vi "http connection handler.vi"(8 "http responder":refnum<class "http responder.lvclass">, 9 "remote address":string, 10 "basic HTTP handler dataset":refnum<class "basic HTTP handler dataset.lvclass">, 11 "connection":refnum<k5>) -> ()   [LabVIEW 2016, in "Basic HTTP server.lvclass"]
uses:
  Basic HTTP server.lvclass
  HTTP responder/http responder.lvclass
  HTTP handler dataset/basic HTTP handler dataset.lvclass
  http request.ctl
  http method.ctl
  HTTP headers/http header data.ctl
  http response.ctl
  http response packet type.ctl
  HTTP handler dataset/basic HTTP handler dataset.lvclass/basic HTTP handler dataset.ctl
  http parse state.ctl
  HTTP headers/http headers.lvlib
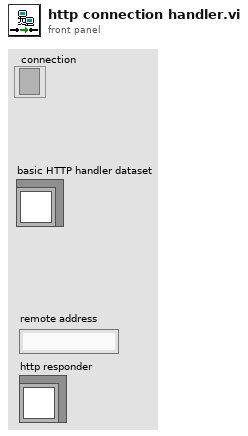
[diagram p1: front panel]
types:
  T1 = typedef "Basic HTTP server.lvclass/http response.ctl" = cluster{"packet type":T2, "reason code":u16, "status string":string, "headers":T3, "cookies":string[], "data":string}
  T2 = typedef "Basic HTTP server.lvclass/http response packet type.ctl" = enum16{"full response", "header only", "data only", "last data", "raw output"}
  T3 = typedef "http headers.lvlib/http header data.ctl" = cluster{"lookup":variant}
  T4 = typedef "Basic HTTP server.lvclass/http request.ctl" = cluster{"type":T5, "remote address":string, "method":string, "url":string, "version":string, "headers":T3, "data":string}
  T5 = typedef "Basic HTTP server.lvclass/http method.ctl" = enum16{"application", "error", "upgrade", "expect"}
  T6 = typedef "Basic HTTP server.lvclass/http server info.ctl" = cluster{"port":u16}
  T7 = typedef "Basic HTTP server.lvclass/http server properties.ctl" = cluster{"max url size":i32, "max header":i32, "timeout ms":i32, "max data size":i32}
  T8 = typedef "Basic HTTP server.lvclass/http parse state.ctl" = enum16{"function", "headers", "data"}
  T9 = enum16{"Standard", "Buffered", "CRLF", "Immediate"}
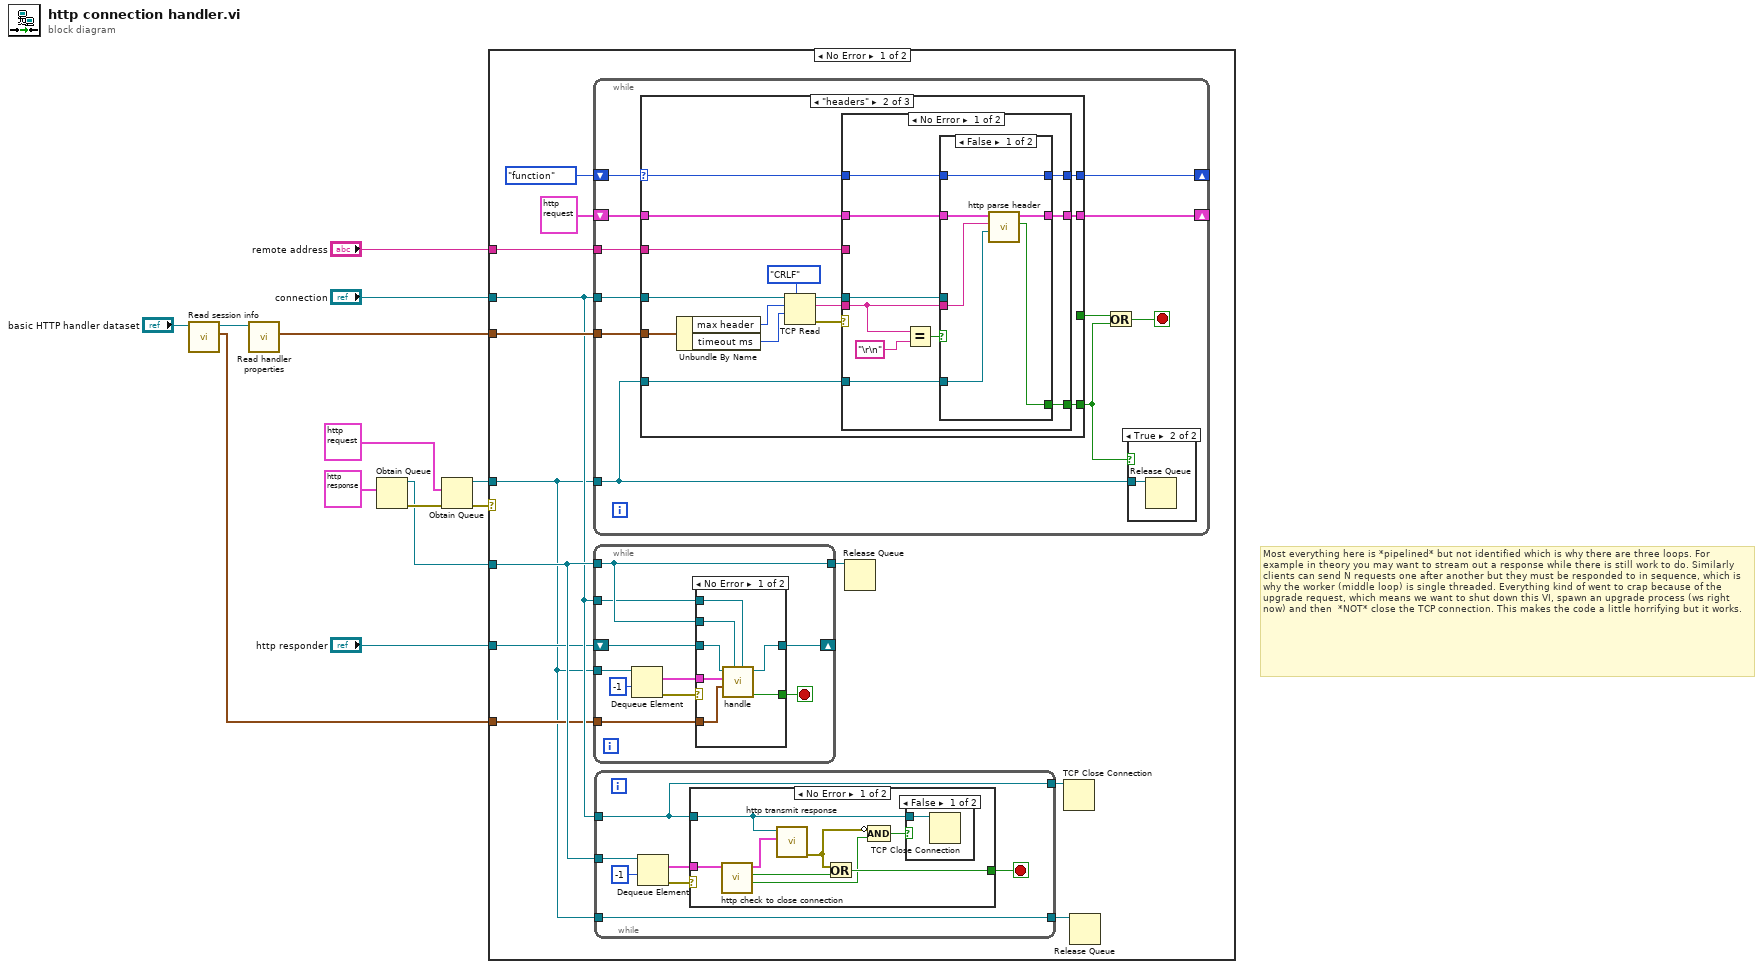
[diagram p0: block diagram]
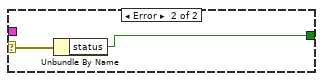
[diagram p3: hidden frame]
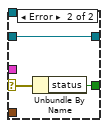
[diagram p4: hidden frame]
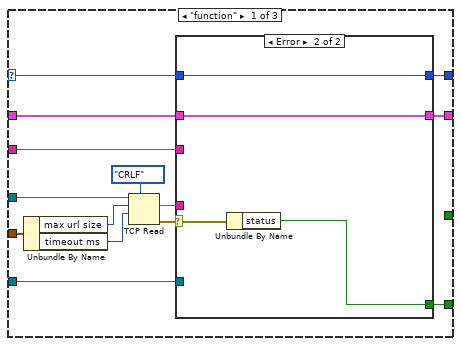
[diagram p6: hidden frame]
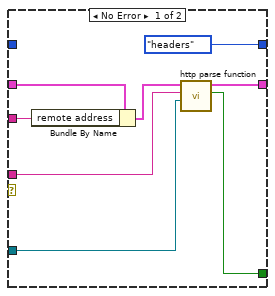
[diagram p7: hidden frame]
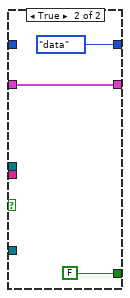
[diagram p8: hidden frame]
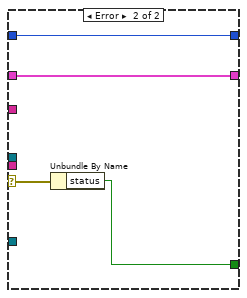
[diagram p9: hidden frame]
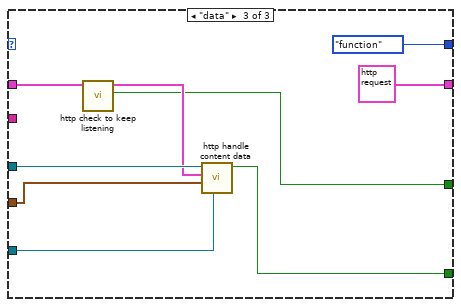
[diagram p10: hidden frame]
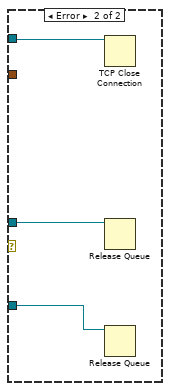
[diagram p11: hidden frame]
diagram:
  # "Most everything here is *pipelined* but not identified which is why there are three loops. For example in theory you may want to stream out a response while there is still work to do. Similarly clients can send N requests one after another but they must be responded to in sequence, which is why the worker (middle loop) is single threaded. Everything kind of went to crap because of the upgrade request, which means we want to shut down this VI, spawn an upgrade process (ws right now) and then  *NOT* close the TCP connection. This makes the code a little horrifying but it works."
  n1 = call "Read session info.vi"("basic HTTP handler dataset in"="basic HTTP handler dataset") -> ("server information"=w1:T6, "basic HTTP handler dataset out"=w2:refnum<class "basic HTTP handler dataset.lvclass">)  [unwired: 9 in]
  n2 = call "Read handler properties.vi"("basic HTTP handler dataset in"=w2) -> ("server properties"=w4:T7)  [unwired: 9 in, 1 out]
  n3 = Obtain Queue(element data type=T1 {"packet type"=enum."full response", "reason code"=0, "status string"="", "headers"={"lookup"=variant}, "cookies"=[], "data"=""} ("application request")) -> (queue out=w6:refnum<queue>, error out=w10:errorcluster)  [unwired: 4 in, 1 out]
  n4 = Obtain Queue(element data type=T4 {"type"=enum."application", "remote address"="", "method"="", "url"="", "version"="", "headers"={"lookup"=variant}, "data"=""} ("application request"), error in (no error)=w10) -> (queue out=w7:refnum<queue>, error out=w12:errorcluster)  [unwired: 3 in, 1 out]
  n5 = case shown="No Error" w12 {
    tunnel: "connection" -> [w20 w151]
    tunnel: "remote address" -> [w25 _]
    tunnel: w7 -> [w16 w150]
    tunnel: w4 -> [w23 _]
    tunnel: w6 -> [w21 w149]
    tunnel: "http responder" -> [w18 _]
    tunnel: w1 -> [w17 _]
    frame No Error {
      n6 = while {
        tunnel: w20 -> [w64]
        shift-right: [w73] -> _
        shift-left: T4 {"type"=enum."application", "remote address"="", "method"="", "url"="", "version"="", "headers"={"lookup"=variant}, "data"=""} ("application request") -> [w74]
        tunnel: w16 -> [w66]
        shift-right: [w72] -> _
        shift-left: http_parse_state."function" -> [w69]
        tunnel: w25 -> [w71]
        tunnel: w23 -> [w70]
        stop <- w68 stop-if-true
        n7 = case shown="\"headers\"" w69 {
          selector: w69 -> [w80 w105 _]
          tunnel: w74 -> [w89 w116 w142]
          tunnel: [w88 w115 T4 {"type"=enum."application", "remote address"="", "method"="", "url"="", "version"="", "headers"={"lookup"=variant}, "data"=""} ("application request")] -> w73
          tunnel: w64 -> [w85 w112 w145]
          tunnel: [w83 w110 http_parse_state."function"] -> w72
          tunnel: [w82 w109 w146] -> w67
          tunnel: w71 -> [w81 w107 _]
          tunnel: w66 -> [w76 w106 w143]
          tunnel: w70 -> [w79 w104 w144]
          tunnel: [_ _ w140] -> w65
          frame "function" {
            n8 = Unbundle By Name(w79) -> ("max url size"=w78:i32, "timeout ms"=w77:i32)
            n9 = TCP Read(connection ID=w85, bytes to read=w78, 7:T9."CRLF" ("mode (standard)"), 9:w77) -> (data out=w84:string, error out=w86:errorcluster)  [unwired: 1 in, 1 out]
            n10 = case shown="Error" w86 {
              selector: w86 -> [_ w100]
              tunnel: w89 -> [w94 w101]
              tunnel: [w95 w101] -> w88
              tunnel: [w93 w98] -> w82
              tunnel: w84 -> [w97 _]
              tunnel: w80 -> [_ w99]
              tunnel: [http_parse_state."headers" w99] -> w83
              tunnel: w81 -> [w92 _]
              tunnel: w76 -> [w90 _]
              frame No Error {
                n11 = Bundle By Name(cluster=w94, "remote address"=w92) -> (w91:T4)
                n12 = call "http parse function.vi"("handler queue"=w90, "data in"=w97, "application request in"=w91) -> ("abort"=w93:bool, "application request out"=w95:T4)  [unwired: 7 in]
              }
              frame Error {
                n13 = Unbundle By Name(w100) -> ("status"=w98:bool)
              }
            }
          }
          frame "headers" {
            n14 = Unbundle By Name(w104) -> ("max header"=w103:i32, "timeout ms"=w102:i32)
            n15 = TCP Read(connection ID=w112, bytes to read=w103, 7:T9."CRLF" ("mode (standard)"), 9:w102) -> (connection ID out=w108:refnum<k5>, data out=w111:string, error out=w113:errorcluster)  [unwired: 1 in]
            n16 = case shown="No Error" w113 {
              selector: w113 -> [_ w138]
              tunnel: w116 -> [w122 w139]
              tunnel: [w123 w139] -> w115
              tunnel: [w121 w136] -> w109
              tunnel: w106 -> [w117 _]
              tunnel: w111 -> [w125 _]
              tunnel: w105 -> [w126 w137]
              tunnel: [w124 w137] -> w110
              tunnel: w108 -> [w120 _]
              tunnel: w107 -> [_ _]
              frame No Error {
                n17 = Equal?(x=w125, y="\r\n" ("x")) -> (x = y?=w118:bool)
                n18 = case shown="False" w118 {
                  tunnel: w125 -> [w131 _]
                  tunnel: w122 -> [w130 w134]
                  tunnel: [w129 w134] -> w123
                  tunnel: w126 -> [w132 _]
                  tunnel: [w132 http_parse_state."data"] -> w124
                  tunnel: [w128 FALSE ("abort")] -> w121
                  tunnel: w120 -> [_ _]
                  tunnel: w117 -> [w127 _]
                  frame False {
                    n19 = call "http parse header.vi"("handler queue"=w127, "data in"=w131, "application request"=w130) -> ("abort"=w128:bool, "application request out"=w129:T4)  [unwired: 7 in]
                  }
                  frame True {
                  }
                }
              }
              frame Error {
                n20 = Unbundle By Name(w138) -> ("status"=w136:bool)
              }
            }
          }
          frame "data" {
            n21 = call "http check to keep listening.vi"("application request in"=w142) -> ("stop listening"=w140:bool, "application request out"=w141:T4)  [unwired: 9 in]
            n22 = call "http handle content data.vi"("exec queue"=w143, "server properties"=w144, "application request"=w141, "TCP Network Connection in"=w145) -> ("abort"=w146:bool)  [unwired: 7 in]
          }
        }
        n23 = Or(x=w65, y=w67) -> (x .or. y?=w68:bool)
        n24 = case shown="True" w67 {
          tunnel: w66 -> [_ w75]
          frame False {
          }
          frame True {
            n25 = Release Queue(queue=w75) -> ()  [unwired: 2 in, 3 out]
          }
        }
      }
      n26 = while {
        tunnel: w21 -> [w48]
        tunnel: [w48] -> w22
        tunnel: w16 -> [w53]
        tunnel: w20 -> [w47]
        shift-right: [w45] -> _
        shift-left: w18 -> [w46]
        tunnel: w17 -> [w44]
        stop <- w50 stop-if-true
        n27 = Dequeue Element(queue=w53, timeout in ms (-1)=-1) -> (element=w49:T4, error out=w51:errorcluster)  [unwired: 1 in, 2 out]
        n28 = case shown="No Error" w51 {
          selector: w51 -> [_ w63]
          tunnel: [w56 w62] -> w50
          tunnel: w49 -> [w57 _]
          tunnel: w48 -> [w60 _]
          tunnel: w47 -> [w55 _]
          tunnel: w46 -> [w59 w61]
          tunnel: [w58 w61] -> w45
          tunnel: w44 -> [w54 _]
          frame No Error {
            n29 = call "handle.vi"("TCP connection"=w55, "response queue"=w60, "server information"=w54, "application request in"=w57, "http responder in"=w59) -> ("stop processing"=w56:bool, "http responder out"=w58:refnum<class "http responder.lvclass">)  [unwired: 5 in]
          }
          frame Error {
            n30 = Unbundle By Name(w63) -> ("status"=w62:bool)
          }
        }
      }
      n31 = while {
        tunnel: w20 -> [w26]
        tunnel: w21 -> [w32]
        tunnel: [w27] -> w19
        tunnel: w16 -> [w27]
        tunnel: [w26] -> w14
        stop <- w29 stop-if-true
        n32 = Dequeue Element(queue=w32, timeout in ms (-1)=-1) -> (element=w28:T1, error out=w30:errorcluster)  [unwired: 1 in, 2 out]
        n33 = case shown="No Error" w30 {
          selector: w30 -> [_ w43]
          tunnel: [w36 w42] -> w29
          tunnel: w28 -> [w40 _]
          tunnel: w26 -> [w37 _]
          frame No Error {
            n34 = call "http check to close connection.vi"("application request"=w40) -> ("leave connection open?"=w34:bool, "stop process?"=w38:bool, "application request out"=w39:T1)  [unwired: 8 in]
            n35 = call "http transmit response.vi"("application request"=w39, "tcp connection"=w37) -> ("error out"=w33:errorcluster)  [unwired: 9 in]
            n36 = Or(x=w33, y=w38) -> (x .or. y?=w36:bool)
            n37 = Compound Arithmetic op=AND(invert w33, w34) -> (w35:bool)
            n38 = case shown="False" w35 {
              tunnel: w37 -> [w41 _]
              frame False {
                n39 = TCP Close Connection(connection ID=w41) -> ()  [unwired: 2 in, 2 out]
              }
              frame True {
              }
            }
          }
          frame Error {
            n40 = Unbundle By Name(w43) -> ("status"=w42:bool)
          }
        }
      }
      n41 = Release Queue(queue=w22) -> ()  [unwired: 2 in, 3 out]
      n42 = TCP Close Connection(connection ID=w14) -> ()  [unwired: 2 in, 2 out]
      n43 = Release Queue(queue=w19) -> ()  [unwired: 2 in, 3 out]
    }
    frame Error {
      n44 = TCP Close Connection(connection ID=w151) -> ()  [unwired: 2 in, 2 out]
      n45 = Release Queue(queue=w150) -> ()  [unwired: 2 in, 3 out]
      n46 = Release Queue(queue=w149) -> ()  [unwired: 2 in, 3 out]
    }
  }
